vi "Run Process.vi"(8 "error in (no error)":errorcluster, 11 "ChartProc in":refnum<class "ChartProc.lvclass">) -> (0 "error out":errorcluster, 3 "ChartProc out":refnum<class "ChartProc.lvclass">)   [LabVIEW 2020, in "LAF2024Q2.lvlib" / "ChartProc.lvclass"]
uses:
  ChartProc.lvclass
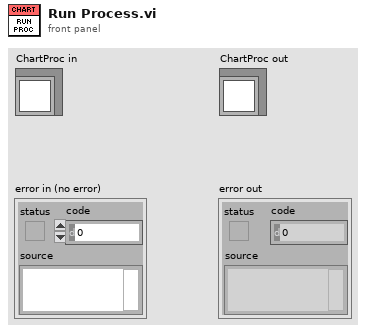
[diagram p1: front panel]
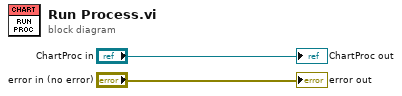
[diagram p0: block diagram]
diagram:
  "error out" <- "error in (no error)"
  "ChartProc out" <- "ChartProc in"
